vi "xcorr_trigger.vi"(10 "enable":bool, 11 "Pulse width":u16) -> (3 "trigger":bool)   [LabVIEW 2017]
uses:
  <instrlib>/_niInstr/Basic Elements/v1/FPGA/niInstr Basic Elements v1 FPGA.lvlib
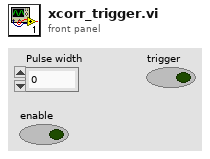
[diagram p1: front panel]
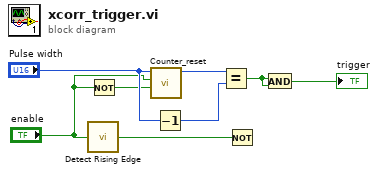
[diagram p0: block diagram]
diagram:
  n1 = call <instrlib>:"Detect Rising Edge.vi"("signal"="enable") -> ("edge detected"=w8:bool)  [unwired: 14 in]
  n2 = Not(x="enable") -> (.not. x?=w3:bool)
  n3 = call "Counter_reset.vi"("reset"=w3, "enable"="enable", "limit"="Pulse width") -> ("count"=w5:u16)  [unwired: 8 in]
  n4 = Decrement(x="Pulse width") -> (x-1=w4:u16)
  n5 = Equal?(x=w5, y=w4) -> (x = y?=w1:bool)
  n6 = Not(x=w8) -> ()  [unwired: 1 out]
  n7 = And(x=w1, y=w1) -> (x .and. y?=→"trigger":bool)
